vi "Scripting_CleanUpControls.vi"(8 "error in (no error)":errorcluster, 11 "VI-Path/VI-Ref":variant) -> (0 "error out":errorcluster, 3 "ViRef":refnum<vi>)   [LabVIEW 2020]
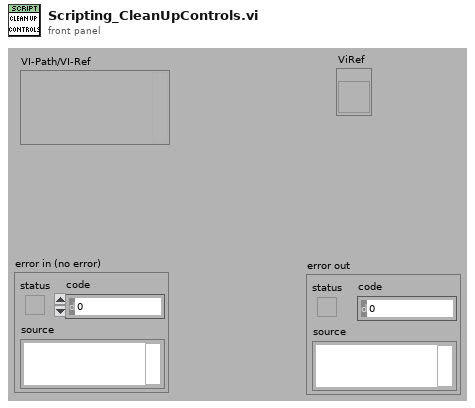
[diagram p1: front panel]
types:
  T1 = typedef "LVRectTypeDef.ctl" = cluster{"Left":i16, "Top":i16, "Right":i16, "Bottom":i16}
  T2 = typedef "LVPositionTypeDef.ctl" = cluster{"Left":i32, "Top":i32}
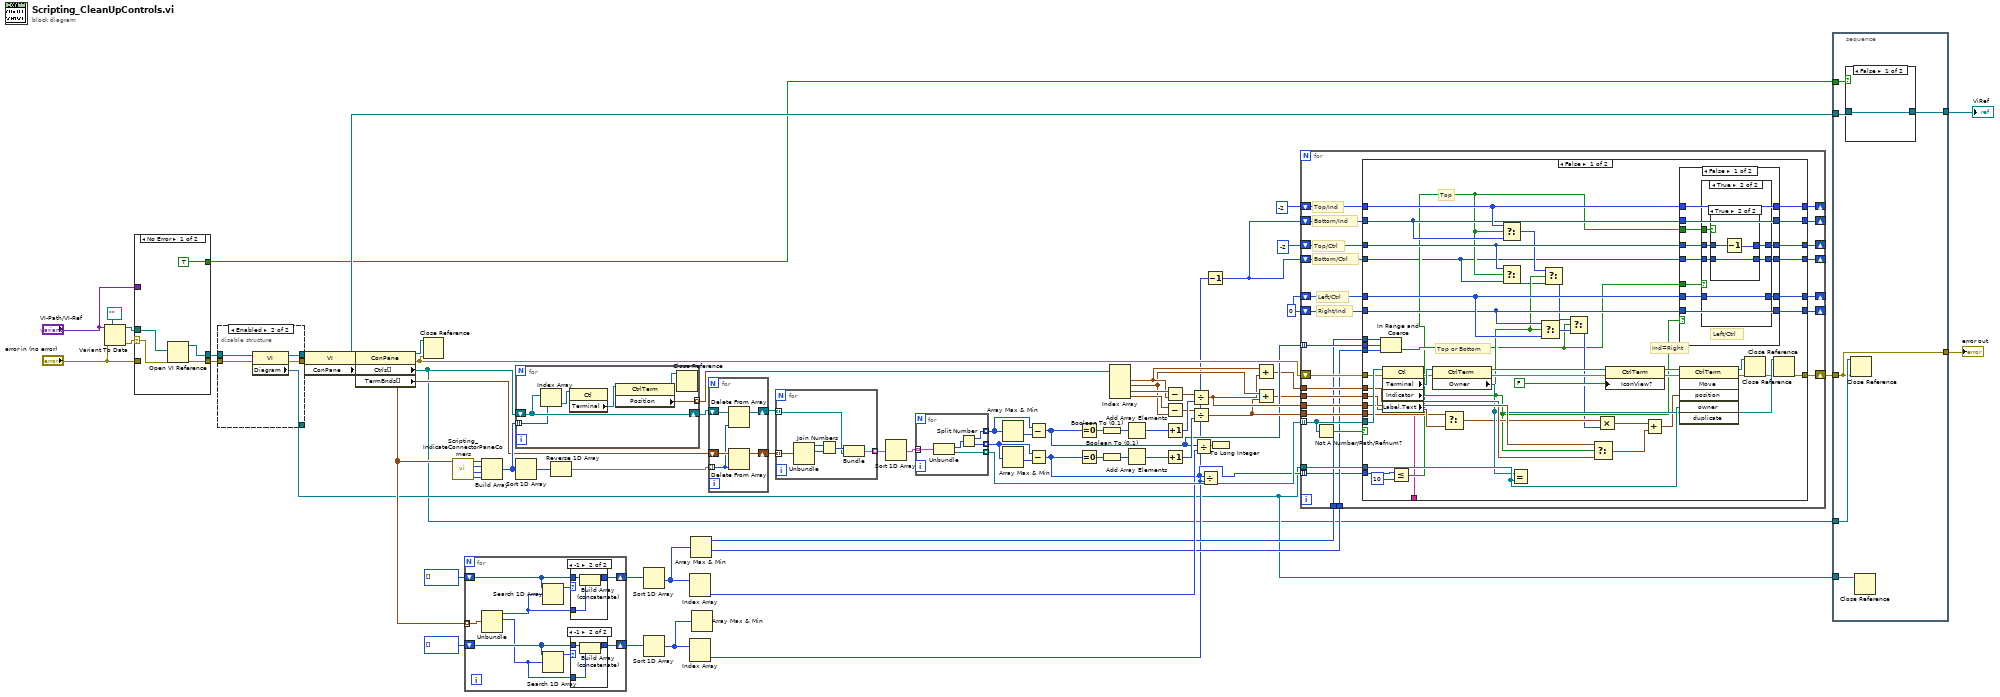
[diagram p0: block diagram]
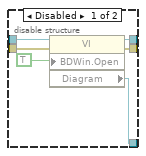
[diagram p2: hidden frame]
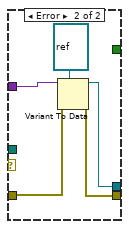
[diagram p3: hidden frame]
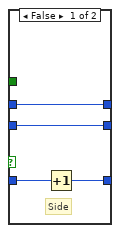
[diagram p4: hidden frame]
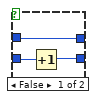
[diagram p5: hidden frame]
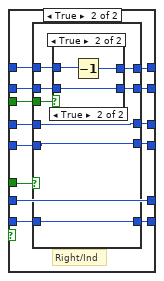
[diagram p6: hidden frame]
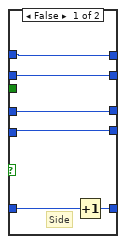
[diagram p7: hidden frame]
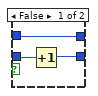
[diagram p8: hidden frame]
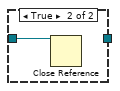
[diagram p12: hidden frame]
diagram:
  w13 = 0 ("Left")
  n1 = Variant To Data(error in="error in (no error)", type=path "" ("vi path"), Variant="VI-Path/VI-Ref") -> (data=w9:path, error out=w8:errorcluster)
  n2 = case shown="No Error" w8 {
    selector: w8 -> [w76 _]
    tunnel: [w77 w82] -> w74
    tunnel: "error in (no error)" -> [_ w80]
    tunnel: [w79 w81] -> w71
    tunnel: w9 -> [w78 _]
    tunnel: "VI-Path/VI-Ref" -> [_ w84]
    tunnel: [TRUE _] -> w4
    frame No Error {
      n3 = Open VI Reference(vi path=w78, error in (no error)=w76) -> (vi reference=w77:refnum<vi>, error out=w79:errorcluster)  [unwired: 4 in]
    }
    frame Error {
      n4 = Variant To Data(error in=w80, type=refnum<vi> refnum ("reference"), Variant=w84) -> (data=w82:refnum<vi>, error out=w81:errorcluster)
    }
  }
  n5 = disable-structure shown="Enabled" {
    disable-tunnel: w74 -> [w90 w95]
    disable-tunnel: [w89 w94] -> w73
    disable-tunnel: w71 -> [w87 w93]
    disable-tunnel: [w86 w92] -> w70
    disable-tunnel: [w85 w91] -> w3
    frame Disabled {
      n6 = property class="VI"(reference=w90, error in=w87, "BDWin.Open"=TRUE ("Block Diagram Window:Open")) -> (reference out=w89:refnum<vi>, error out=w86:errorcluster, "Diagram"=w85:refnum<vi>)
    }
    frame Enabled {
      n7 = property class="VI"(reference=w95, error in=w93) -> (reference out=w94:refnum<vi>, error out=w92:errorcluster, "Diagram"=w91:refnum<vi>)
    }
  }
  n8 = property class="VI"(reference=w73, error in=w70) -> (reference out=w5:refnum<vi>, error out=w69:errorcluster, "ConPane"=w72:refnum<vi>)
  n9 = property class="ConPane"(reference=w72, error in=w69) -> (reference out=w68:refnum<vi>, error out=w47:errorcluster, "Ctrls[]"=w2:refnum<vi>[], "TermBnds[]"=w30:T1[])
  n10 = Close Reference(reference=w68, error in (no error)=w47) -> ()  [unwired: 1 out]
  n11 = call <resource>:"Scripting_IndicateConnectorPaneCorners.vi"("TermBnds[]"=w30) -> ("RightLower"=w56:i32, "LeftLower"=w57:i32, "RightTop"=w58:i32, "LeftTop"=w59:i32)  [unwired: 7 in]
  n12 = for {
    tunnel: w30 -> [w104] mode=indexing
    shift-right: [w101] -> w28
    shift-left: i16[] [] -> [w102]
    shift-right: [w99] -> w27
    shift-left: i16[] [] -> [w98]
    n13 = Unbundle(w104) -> ("Left"=w100:i16, "Top"=w96:i16)  [unwired: 2 out]
    n14 = Search 1D Array(1D array=w102, element=w100) -> (index of element=w103:i32)  [unwired: 1 in]
    n15 = Search 1D Array(1D array=w98, element=w96) -> (index of element=w97:i32)  [unwired: 1 in]
    n16 = case shown="-1" w103 {
      tunnel: w102 -> [w109 w112]
      tunnel: [w109 w111] -> w101
      tunnel: w100 -> [_ w110]
      frame 0, Default {
      }
      frame -1 {
        n17 = Build Array (concatenate)(w112, w110) -> (w111:i16[])
      }
    }
    n18 = case shown="-1" w97 {
      tunnel: w98 -> [w105 w108]
      tunnel: [w105 w107] -> w99
      tunnel: w96 -> [_ w106]
      frame 0, Default {
      }
      frame -1 {
        n19 = Build Array (concatenate)(w108, w106) -> (w107:i16[])
      }
    }
  }
  n20 = Build Array(w59, w58, w57, w56) -> (w49:i32[])
  n21 = for {
    shift-right: [w118] -> w50
    shift-left: w2 -> [w118]
    tunnel: w49 -> [w117] mode=indexing
    tunnel: [w114] -> w48 mode=indexing
    n22 = Index Array(array=w118, index=w117) -> (element=w116:refnum<vi>)
    n23 = property class="Ctl"(reference=w116) -> ("Terminal"=w115:refnum<vi>)  [unwired: 1 in, 2 out]
    n24 = property class="CtrlTerm"(reference=w115) -> (reference out=w113:refnum<vi>, "Position"=w114:T2)  [unwired: 1 in, 1 out]
    n25 = Close Reference(reference=w113) -> ()  [unwired: 1 in, 1 out]
  }
  n26 = Sort 1D Array(array=w49) -> (sorted array=w55:i32[])
  n27 = Reverse 1D Array(array=w55) -> (reversed array=w54:i32[])
  n28 = Sort 1D Array(array=w28) -> (sorted array=w23:i16[])
  n29 = Sort 1D Array(array=w27) -> (sorted array=w20:i16[])
  n30 = Index Array(array=w23) -> (element #2=w25:i16)  [unwired: 2 in, 1 out]
  n31 = Index Array(array=w20) -> (element #2=w17:i16)  [unwired: 2 in, 1 out]
  n32 = Array Max & Min(array=w23) -> (max value=w22:i16, min value=w21:i16)  [unwired: 2 out]
  n33 = Array Max & Min(array=w20) -> ()  [unwired: 4 out]
  n34 = for {
    shift-right: [w122] -> w53
    shift-left: w50 -> [w123]
    tunnel: w54 -> [w119] mode=indexing
    shift-right: [w121] -> w52
    shift-left: w30 -> [w120]
    n35 = Delete From Array(array=w123, index=w119) -> (array with subset deleted=w122:refnum<vi>[])  [unwired: 1 in, 1 out]
    n36 = Delete From Array(array=w120, index=w119) -> (array with subset deleted=w121:T1[])  [unwired: 1 in, 1 out]
  }
  n37 = for {
    tunnel: [w126] -> w65 mode=indexing
    tunnel: w52 -> [w125] mode=indexing
    tunnel: w53 -> [w124] mode=indexing
    n38 = Unbundle(w125) -> ("Left"=w129:i16, "Top"=w128:i16)  [unwired: 2 out]
    n39 = Join Numbers(hi=w129, lo=w128) -> ((hi.lo)=w127:u32)
    n40 = Bundle(w127, w124) -> (w126:cluster{u32, refnum<vi>})  [unwired: 1 in]
  }
  n41 = Sort 1D Array(array=w65) -> (sorted array=w64:cluster{u32, refnum<vi>}[])
  n42 = for {
    tunnel: w64 -> [w134] mode=indexing
    tunnel: [w133] -> w51 mode=indexing
    tunnel: [w131] -> w63 mode=indexing
    tunnel: [w130] -> w61 mode=indexing
    n43 = Unbundle(w134) -> (w132:u32, w133:refnum<vi>)
    n44 = Split Number(x=w132) -> (hi(x)=w131:u16, lo(x)=w130:u16)
  }
  n45 = Array Max & Min(array=w63) -> (min value=w62:u16)  [unwired: 3 out]
  n46 = Array Max & Min(array=w61) -> (min value=w60:u16)  [unwired: 3 out]
  n47 = Subtract(x=w63, y=w62) -> (x-y=w18:u16[])
  n48 = Subtract(x=w61, y=w60) -> (x-y=w19:u16[])
  n49 = Equal To 0?(x=w18) -> (x = 0?=w43:bool[])
  n50 = Equal To 0?(x=w19) -> (x = 0?=w34:bool[])
  n51 = Boolean To (0,1)(Boolean=w43) -> (0, 1=w42:i16[])
  n52 = Boolean To (0,1)(Boolean=w34) -> (0, 1=w35:i16[])
  n53 = Index Array(array=w48) -> (element #1=w45:T2, element #2=w37:T2, element #3=w46:T2, element #4=w38:T2)  [unwired: 4 in]
  n54 = Add Array Elements(numeric array=w42) -> (sum=w41:i16)
  n55 = Add Array Elements(numeric array=w35) -> (sum=w36:i16)
  n56 = Subtract(x=w46, y=w45) -> (x-y=w44:T2)
  n57 = Subtract(x=w38, y=w37) -> (x-y=w39:T2)
  n58 = Increment(x=w41) -> (x+1=w40:i16)
  n59 = Increment(x=w36) -> (x+1=w33:i16)
  n60 = Divide(x=w44, y=w40) -> (x/y=w32:cluster{"Left":dbl, "Top":dbl})
  n61 = Divide(x=w39, y=w33) -> (x/y=w31:cluster{"Left":dbl, "Top":dbl})
  n62 = Divide(x=w18, y=w25) -> (x/y=w24:dbl[])
  n63 = Divide(x=w19, y=w17) -> ()  [unwired: 1 out]
  n64 = Decrement(x=w17) -> (x-1=w16:i16)
  n65 = To Long Integer(number=w24) -> ()  [unwired: 1 out]
  n66 = Add(x=w45, y=w32) -> (x+y=w14:cluster{"Left":dbl, "Top":dbl})
  n67 = Add(x=w37, y=w31) -> (x+y=w15:cluster{"Left":dbl, "Top":dbl})
  n68 = for {
    shift-right: [w157] -> _
    shift-left: w13 -> [w158]
    tunnel: w51 -> [w156] mode=indexing
    tunnel: w3 -> [w155]
    tunnel: w15 -> [w154]
    tunnel: w14 -> [w153]
    shift-right: [w152] -> _
    shift-left: w13 -> [w151]
    shift-right: [w149] -> w67
    shift-left: w47 -> [w150]
    tunnel: w32 -> [w148]
    tunnel: w31 -> [w147]
    shift-right: [w144] -> _
    shift-left: -2 ("Left") -> [w143]
    shift-right: [w145] -> _
    shift-left: w16 -> [w146]
    shift-right: [w141] -> _
    shift-left: -2 ("Left") -> [w142]
    shift-right: [w140] -> _
    shift-left: w16 -> [w139]
    tunnel: w18 -> [w138] mode=indexing
    tunnel: w22 -> [w137]
    tunnel: w21 -> [w136]
    tunnel: w19 -> [w135] mode=indexing
    # "Bottom/Ind"
    # "Top/Ind"
    # "Bottom/Ctrl"
    # "Top/Ctrl"
    # "Right/Ind"
    # "Left/Ctrl"
    n69 = Not A Number/Path/Refnum?(number/path/refnum=w156) -> (NaN/Path/Refnum?=w159:bool)
    n70 = case shown="False" w159 {
      tunnel: w158 -> [w207 w275]
      tunnel: [w206 w275] -> w157
      tunnel: w156 -> [w204 _]
      tunnel: w155 -> [w203 _]
      tunnel: w154 -> [w202 _]
      tunnel: w153 -> [w201 _]
      tunnel: w151 -> [w198 w274]
      tunnel: [w199 w274] -> w152
      tunnel: w150 -> [w197 w273]
      tunnel: [w194 w273] -> w149
      tunnel: w148 -> [w191 _]
      tunnel: w147 -> [w190 _]
      tunnel: w143 -> [w175 w270]
      tunnel: [w180 w270] -> w144
      tunnel: w146 -> [w160 w269]
      tunnel: [w181 w269] -> w145
      tunnel: w142 -> [w177 w272]
      tunnel: [w179 w272] -> w141
      tunnel: w139 -> [w176 w271]
      tunnel: [w178 w271] -> w140
      tunnel: w138 -> [w167 _]
      tunnel: w137 -> [w166 _]
      tunnel: w136 -> [w165 _]
      tunnel: w135 -> [w164 _]
      tunnel: [w161 _] -> _
      frame False {
        # "Top"
        # "Top or Bottom"
        # "Ind=Right"
        n71 = In Range and Coerce(upper limit=w166, x=w167, lower limit=w165) -> (In Range?=w168:bool)  [unwired: 1 out]
        n72 = property class="Ctl"(reference=w204, error in=w197) -> (error out=w196:errorcluster, "Terminal"=w208:refnum<vi>, "Indicator"=w174:bool, "Label.Text"=w161:string)  [unwired: 1 out]
        n73 = Less Or Equal?(x=w164, y=10) -> (x <= y?=w162:bool)
        n74 = property class="CtrlTerm"(reference=w208, error in=w196) -> (reference out=w205:refnum<vi>, error out=w195:errorcluster, "Owner"=w193:refnum<vi>)
        n75 = Select(t=w190, s=w174, f=w191) -> (s? t:f=w192:cluster{"Left":dbl, "Top":dbl})
        n76 = Select(t=w177, s=w162, f=w176) -> (s? t:f=w173:i32)
        n77 = Select(t=w175, s=w162, f=w160) -> (s? t:f=w172:i32)
        n78 = Equal?(x=w193, y=w203) -> ()  [unwired: 1 out]
        n79 = Select(t=w198, s=w174, f=w207) -> (s? t:f=w171:i32)
        n80 = Select(t=w173, s=w174, f=w172) -> (s? t:f=w170:i32)
        n81 = Select(t=w170, s=w168, f=w171) -> (s? t:f=w169:i32)
        n82 = Select(t=w202, s=w174, f=w201) -> (s? t:f=w200:cluster{"Left":dbl, "Top":dbl})
        n83 = Multiply(x=w192, y=w169) -> (x*y=w188:cluster{"Left":dbl, "Top":dbl})
        n84 = property class="CtrlTerm"(reference=w205, error in=w195, "IconView?"=FALSE ("Icon View?")) -> (reference out=w187:refnum<vi>, error out=w185:errorcluster)
        n85 = Add(x=w188, y=w200) -> (x+y=w189:cluster{"Left":dbl, "Top":dbl})
        n86 = invoke class="CtrlTerm" method="Move"(reference=w187, error in=w185, "position"=w189, "owner"=w203) -> (reference out=w183:refnum<vi>, error out=w184:errorcluster)  [unwired: 2 in, 4 out]
        n87 = case shown="False" w174 {
          tunnel: w207 -> [w219 w248]
          tunnel: [w218 w248] -> w206
          tunnel: w198 -> [w217 w247]
          tunnel: [w217 w246] -> w199
          tunnel: w175 -> [w215 w239]
          tunnel: [w216 w237] -> w180
          tunnel: w160 -> [w210 w238]
          tunnel: [w209 w236] -> w181
          tunnel: w168 -> [w214 w245]
          tunnel: w177 -> [w213 w243]
          tunnel: [w213 w242] -> w179
          tunnel: w176 -> [w212 w241]
          tunnel: [w212 w240] -> w178
          tunnel: w162 -> [w211 w244]
          frame False {
            # "Left/Ctrl"
            n88 = case shown="True" w214 {
              tunnel: w219 -> [w223 w229]
              tunnel: [w222 w229] -> w218
              tunnel: [w221 w225] -> w216
              tunnel: w215 -> [w221 w227]
              tunnel: w211 -> [_ w228]
              tunnel: w210 -> [w220 w226]
              tunnel: [w220 w224] -> w209
              frame False {
                # "Side"
                n89 = Increment(x=w223) -> (x+1=w222:i32)
              }
              frame True {
                n90 = case shown="True" w228 {
                  tunnel: w227 -> [w232 w235]
                  tunnel: [w232 w234] -> w225
                  tunnel: [w231 w233] -> w224
                  tunnel: w226 -> [w230 w233]
                  frame False {
                    n91 = Increment(x=w230) -> (x+1=w231:i16)
                  }
                  frame True {
                    n92 = Decrement(x=w235) -> (x-1=w234:i32)
                  }
                }
              }
            }
          }
          frame True {
            # "Right/Ind"
            n93 = case shown="True" w245 {
              tunnel: w247 -> [w254 w262]
              tunnel: [w253 w262] -> w246
              tunnel: w244 -> [_ w261]
              tunnel: w243 -> [w252 w260]
              tunnel: [w252 w259] -> w242
              tunnel: w241 -> [w251 w258]
              tunnel: [w251 w257] -> w240
              tunnel: w239 -> [w250 w256]
              tunnel: w238 -> [w249 w255]
              tunnel: [w250 w256] -> w237
              tunnel: [w249 w255] -> w236
              frame False {
                # "Side"
                n94 = Increment(x=w254) -> (x+1=w253:i32)
              }
              frame True {
                n95 = case shown="True" w261 {
                  tunnel: w260 -> [w265 w268]
                  tunnel: [w265 w267] -> w259
                  tunnel: [w264 w266] -> w257
                  tunnel: w258 -> [w263 w266]
                  frame False {
                    n96 = Increment(x=w263) -> (x+1=w264:i16)
                  }
                  frame True {
                    n97 = Decrement(x=w268) -> (x-1=w267:i32)
                  }
                }
              }
            }
          }
        }
        n98 = Close Reference(reference=w183, error in (no error)=w184) -> (error out=w182:errorcluster)
        n99 = Close Reference(reference=w193, error in (no error)=w182) -> (error out=w194:errorcluster)
      }
      frame True {
      }
    }
  }
  n100 = stacked-sequence {
    tunnel: w67 -> [w280]
    tunnel: [w280] -> w66
    tunnel: w2 -> [w281]
    tunnel: w5 -> [w279]
    tunnel: w4 -> [w278]
    tunnel: w3 -> [w277]
    tunnel: [w276] -> w1
    frame #0 {
      n101 = case shown="False" w278 {
        tunnel: w279 -> [w282 w283]
        tunnel: [w282 _] -> w276
        frame False {
        }
        frame True {
          n102 = Close Reference(reference=w283) -> ()  [unwired: 1 in, 1 out]
        }
      }
      n103 = Close Reference(reference=w281, error in (no error)=w280) -> ()  [unwired: 1 out]
      n104 = Close Reference(reference=w277) -> ()  [unwired: 1 in, 1 out]
    }
  }
  "error out" <- w66
  "ViRef" <- w1
